vi "1D Interpolation.vi"() -> ()   [LabVIEW 2014]
doc: "This example shows the operation of the 1D interpolation VI using three selectable test sets."
uses:
  <vilib>/Analysis/1siggen.llb/Ramp Pattern by Delta.vi
  <vilib>/gmath/NI_Gmath.lvlib
  <vilib>/Analysis/NI_AALBase.lvlib
panel:
  in  "Stop":bool
  in  "Tab Control":enum32{"Graph", "Data"}(tab)
  out "1D Interpolation Graph":cluster{"yi":dbl[], "ramp data":dbl[]}[](graph)
  out "Interpolated Data":dbl[][](array[numeric])
  out "Original Data":dbl[][](array[numeric])
  in  "Method":i32(ring)=2 items=["nearest", "linear", "spline", "cubic Hermite", "Lagrange"]
  in  "Data Sets":enum16{"Test Set 1", "Test Set 2", "Test Set 3"}(ring)
  # "Overview: Demonstrates the operation of the Interpolate 1D VI using three selectable test sets.\nRequirements: LabVIEW Full Development System\nInstructions: \n1. Run the VI.\n2. Modify the Data Sets and interpolation Method, and view the results on both the Graph and Data tabs.\n3. Click Stop to stop the VI."
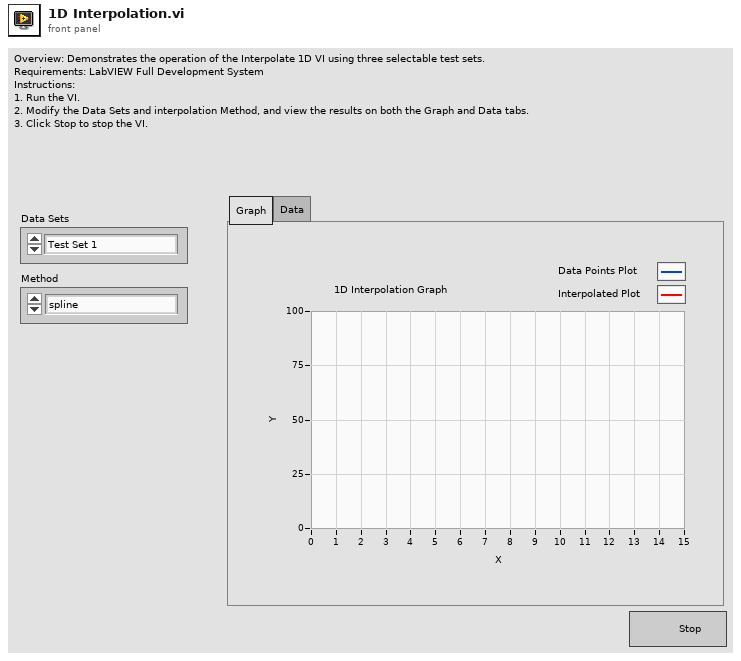
[diagram p1: front panel]
types:
  T1 = cluster{"starting value":dbl, "increment":dbl, "final value":dbl}
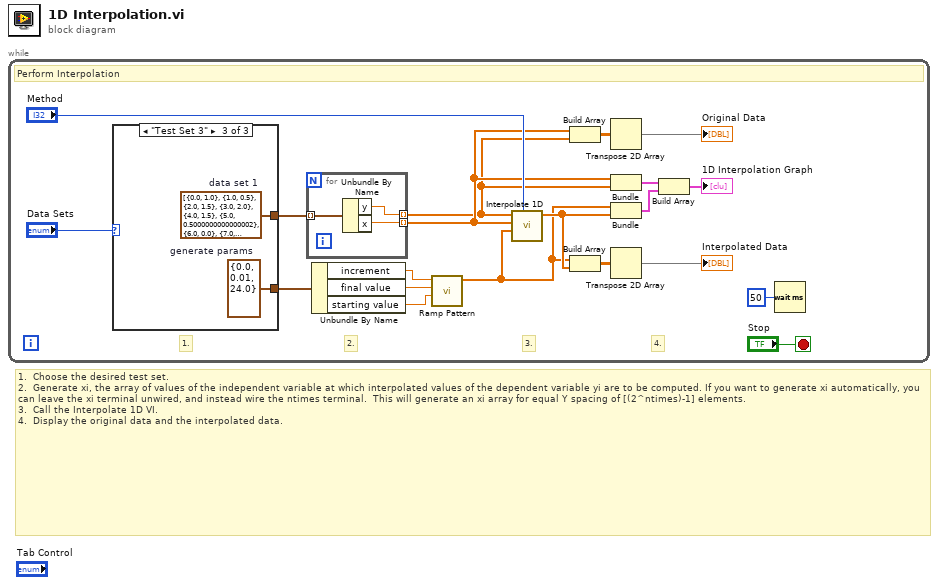
[diagram p0: block diagram]
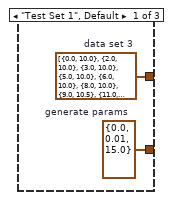
[diagram p2: hidden frame]
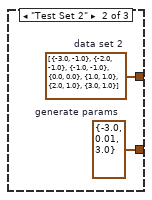
[diagram p3: hidden frame]
diagram:
  # "1.  Choose the desired test set.\n2.  Generate xi, the array of values of the independent variable at which interpolated values of the dependent variable yi are to be computed. If you want to generate xi automatically, you can leave the xi terminal unwired, and instead wire the ntimes terminal.  This will generate an xi array for equal Y spacing of [(2^ntimes)-1] elements.\n3.  Call the Interpolate 1D VI.\n4.  Display the original data and the interpolated data."
  n1 = while {
    stop <- "Stop" stop-if-true
    # "4."
    # "3."
    # "2."
    # "1."
    # "Perform Interpolation"
    n2 = case shown="\"Test Set 3\"" "Data Sets" {
      tunnel: [w25 w27 w29] -> w19
      tunnel: [w24 w26 w28] -> w18
      frame "Test Set 1", Default {
        w24 = T1 {"starting value"=0.0, "increment"=0.01, "final value"=15.0}  # generate params
        w25 = cluster{"x":dbl, "y":dbl}[] [{"x"=0.0, "y"=10.0}, {"x"=2.0, "y"=10.0}, {"x"=3.0, "y"=10.0}, {"x"=5.0, "y"=10.0}, {"x"=6.0, "y"=10.0}, {"x"=8.0, "y"=10.0}, {"x"=9.0, "y"=10.5}, {"x"=11.0, "y"=15.0}, {"x"=12.0, "y"=50.0}, {"x"=14.0, "y"=60.0}, {"x"=15.0, "y"=85.0}]  # data set 3
      }
      frame "Test Set 2" {
        w26 = T1 {"starting value"=-3.0, "increment"=0.01, "final value"=3.0}  # generate params
        w27 = cluster{"x":dbl, "y":dbl}[] [{"x"=-3.0, "y"=-1.0}, {"x"=-2.0, "y"=-1.0}, {"x"=-1.0, "y"=-1.0}, {"x"=0.0, "y"=0.0}, {"x"=1.0, "y"=1.0}, {"x"=2.0, "y"=1.0}, {"x"=3.0, "y"=1.0}]  # data set 2
      }
      frame "Test Set 3" {
        w28 = T1 {"starting value"=0.0, "increment"=0.01, "final value"=24.0}  # generate params
        w29 = cluster{"x":dbl, "y":dbl}[] [{"x"=0.0, "y"=1.0}, {"x"=1.0, "y"=0.5}, {"x"=2.0, "y"=1.5}, {"x"=3.0, "y"=2.0}, {"x"=4.0, "y"=1.5}, {"x"=5.0, "y"=0.5000000000000002}, {"x"=6.0, "y"=0.0}, {"x"=7.0, "y"=0.4999999999999998}, {"x"=8.0, "y"=1.4999999999999998}, {"x"=9.0, "y"=2.0}, {"x"=10.0, "y"=2.0}, {"x"=11.0, "y"=2.0}, {"x"=12.0, "y"=2.0}, {"x"=13.0, "y"=-0.5}, {"x"=14.0, "y"=-0.5}, {"x"=15.0, "y"=2.0}, {"x"=16.0, "y"=0.0}, {"x"=17.0, "y"=0.0}, {"x"=18.0, "y"=0.0}, {"x"=19.0, "y"=0.0}, {"x"=20.0, "y"=1.0}, {"x"=21.0, "y"=0.0}, {"x"=22.0, "y"=0.0}, {"x"=23.0, "y"=0.0}, {"x"=24.0, "y"=2.0}]  # data set 1
      }
    }
    n3 = for {
      tunnel: w19 -> [w23] mode=indexing
      tunnel: [w22] -> w12 mode=indexing
      tunnel: [w21] -> w13 mode=indexing
      n4 = Unbundle By Name(w23) -> ("y"=w22:dbl, "x"=w21:dbl)
    }
    n5 = Unbundle By Name(w18) -> ("increment"=w4:dbl, "final value"=w3:dbl, "starting value"=w2:dbl)
    n6 = call-poly <vilib>:"Ramp Pattern.vi"("start"=w2, "end"=w3, "delta"=w4) -> ("Ramp Pattern"=w5:dbl[])  [unwired: 6 in, 2 out]
    n7 = call <vilib>:"Interpolate 1D.vi"("method"="Method", "xi"=w5, "X"=w13, "Y"=w12) -> ("yi"=w8:dbl[])  [unwired: 5 in, 2 out]
    n8 = Build Array(w13, w12) -> (w11:dbl[][])
    n9 = Build Array(w5, w8) -> (w9:dbl[][])
    n10 = Transpose 2D Array(2D array=w11) -> (transposed array=→"Original Data":dbl[][])
    n11 = Bundle(w13, w12) -> (w16:cluster{dbl[], dbl[]})  [unwired: 1 in]
    n12 = Bundle("Ramp Pattern"=w5, "yi"=w8) -> (w17:cluster{"Ramp Pattern":dbl[], "yi":dbl[]})  [unwired: 1 in]
    n13 = Transpose 2D Array(2D array=w9) -> (transposed array=→"Interpolated Data":dbl[][])
    n14 = Build Array(w16, w17) -> (→"1D Interpolation Graph":cluster{"Ramp Pattern":dbl[], "yi":dbl[]}[])
    n15 = Wait (ms)(milliseconds to wait=u32 50) -> ()  [unwired: 1 out]
  }
